vi "Set Tester Tx.vi"(8 "error in (no error)":errorcluster, 10 "Tester Tx":refnum<vi>, 11 "PLC Sim Controller Actor in":refnum<class "PLC Sim Controller Actor.lvclass">) -> (0 "error out":errorcluster, 3 "PLC Sim Controller Actor out":refnum<class "PLC Sim Controller Actor.lvclass">)   [LabVIEW 2019]
uses:
  PLC Sim Controller Actor.lvclass
  C:/Program Files (x86)/National Instruments/LabVIEW 2019/vi.lib/ActorFramework/Actor/Actor.lvclass
  <vilib>/ActorFramework/Message Enqueuer/Message Enqueuer.lvclass
  Station Actor/Station Actor/Custom Controls/Tester Tx Dataset.ctl
  Station Actor/Station Actor/Station Actor.lvclass
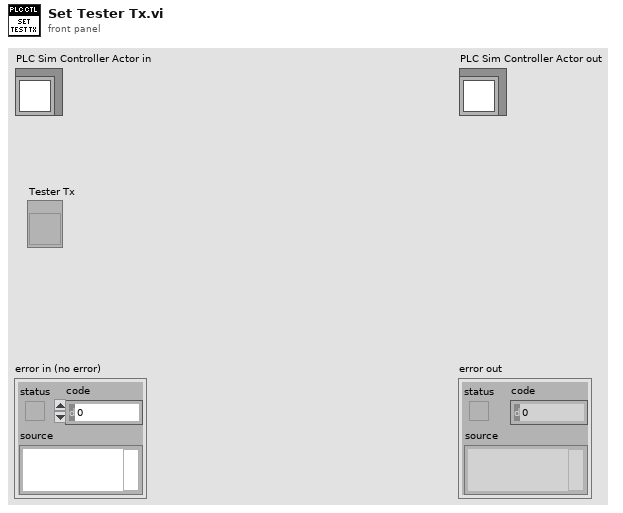
[diagram p1: front panel]
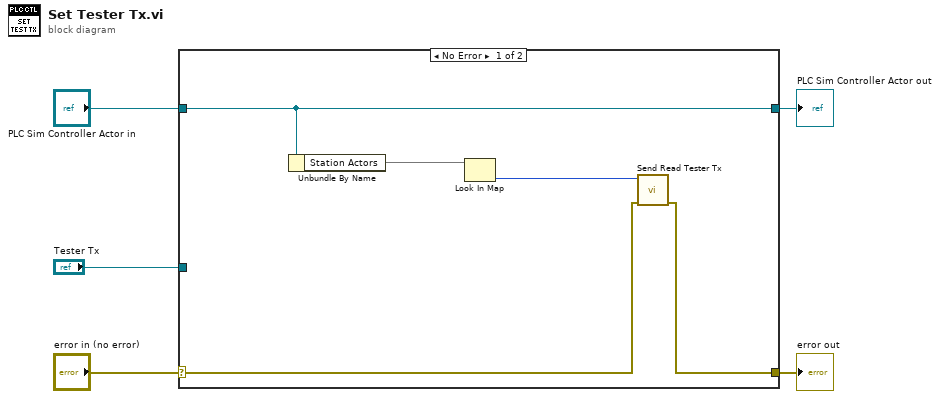
[diagram p0: block diagram]
diagram:
  n1 = case shown="No Error" "error in (no error)" {
    selector: "error in (no error)" -> [w9 w12]
    tunnel: [w8 w12] -> w4
    tunnel: [w10 w11] -> w2
    tunnel: "PLC Sim Controller Actor in" -> [w10 w11]
    tunnel: "Tester Tx" -> [_ _]
    frame No Error {
      n2 = Unbundle By Name(w10) -> ("Station Actors"=w7)
      n3 = Look In Map(map=w7) -> (value=w6:i32)  [unwired: 2 in, 1 out]
      n4 = call "Send Read Tester Tx.vi"("error in (no error)"=w9, "Message Enqueuer"=w6) -> ("error out"=w8:errorcluster)  [unwired: 8 in, 1 out]
    }
    frame Error {
    }
  }
  "error out" <- w4
  "PLC Sim Controller Actor out" <- w2
